vi "Pool Avg.vi"(1 "Input":dbl) -> (0 "Output Avg":dbl)   [LabVIEW 2011]
panel:
  out "Amplitude":dbl
  out "Minimum":dbl
  out "Maximum":dbl
  in  "Sample Size":i32
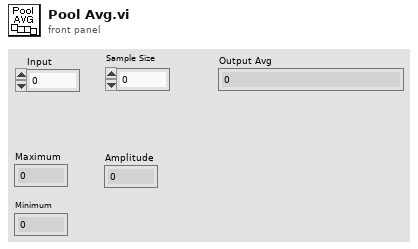
[diagram p1: front panel]
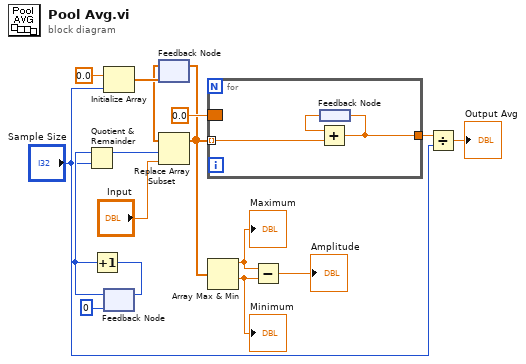
[diagram p0: block diagram]
diagram:
  n1 = Initialize Array(0.0 ("element"), "Sample Size") -> (w15:dbl[])
  n2 = feedback #1(0) -> (w10:i32)
  n3 = Quotient & Remainder(x=w10, y="Sample Size") -> (x-y*floor(x/y)=w9:i32)  [unwired: 1 out]
  n4 = Increment(x=w10) -> (x+1=w11:i32)
  n5 = feedback-in #1(w11) -> ()
  n6 = feedback #2(w15) -> (w14:dbl[])
  n7 = Replace Array Subset(array=w14, new element="Input", index=w9) -> (w1:dbl[])
  n8 = feedback-in #2(w1) -> ()
  n9 = for {
    tunnel: w1 -> [w18] mode=indexing
    tunnel: [w17] -> w8
    border: 0.0 -> [_]
    n10 = feedback #3() -> (w19:dbl)
    n11 = Add(x=w19, y=w18) -> (x+y=w17:dbl)
    n12 = feedback-in #3(w17) -> ()
  }
  n13 = Array Max & Min(array=w1) -> (max value=w4:dbl, min value=w3:dbl)  [unwired: 2 out]
  "Maximum" <- w4
  "Minimum" <- w3
  n14 = Subtract(x=w4, y=w3) -> (x-y=→"Amplitude":dbl)
  n15 = Divide(x=w8, y="Sample Size") -> (x/y=→"Output Avg":dbl)
